vi "fix_ICS_msg.vi"(11 "Msg in":string) -> (3 "JSON":string)   [LabVIEW 2018]
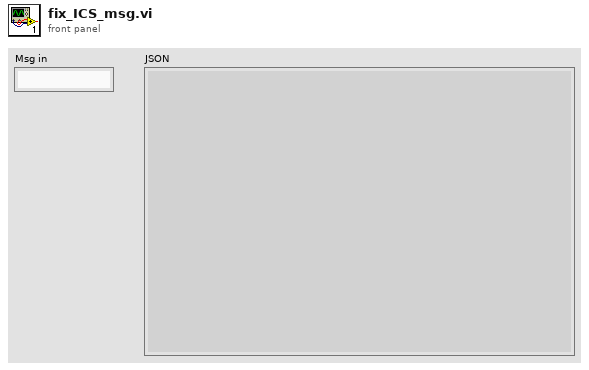
[diagram p1: front panel]
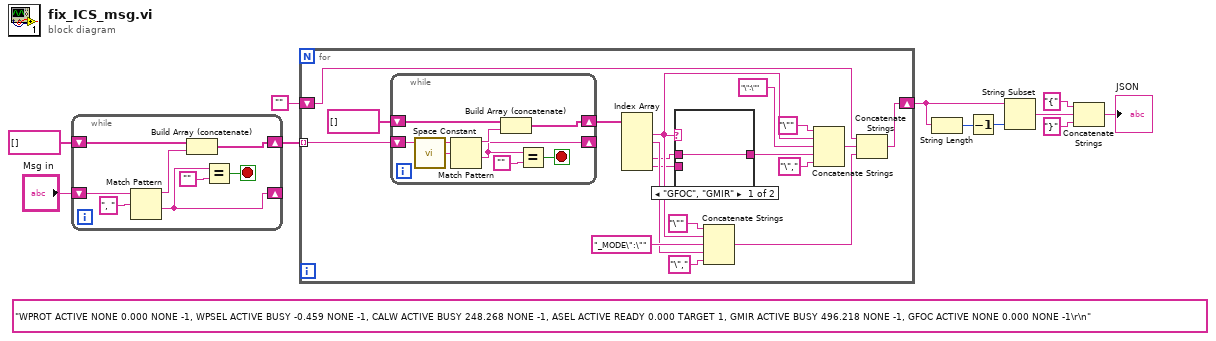
[diagram p0: block diagram]
diagram:
  (unwired) "WPROT ACTIVE NONE 0.000 NONE -1, WPSEL ACTIVE BUSY -0.459 NONE -1, CALW ACTIVE BUSY 248.268 NONE -1, ASEL ACTIVE READY 0.000 TARGET 1, GMIR ACTIVE BUSY 496.218 NONE -1, GFOC ACTIVE NONE 0.000 NONE -1\r\n" ("search string/char (-)")
  n1 = while {
    shift-right: [w16] -> w2
    shift-left: string[] [] -> [w17]
    shift-right: [w12] -> _
    shift-left: "Msg in" -> [w15]
    stop <- w18 stop-if-true
    n2 = Match Pattern(string=w15, regular expression=", " ("search string/char (-)")) -> (before substring=w13:string, after substring=w12:string)  [unwired: 1 in, 2 out]
    n3 = Build Array (concatenate)(w17, w13) -> (w16:string[])
    n4 = Equal?(x=w12, y="") -> (x = y?=w18:bool)
  }
  n5 = for {
    tunnel: w2 -> [w36] mode=indexing
    shift-right: [w25] -> w4
    shift-left: "" -> [w24]
    n6 = while {
      shift-right: [w44] -> w35
      shift-left: string[] [] -> [w45]
      shift-right: [w41] -> _
      shift-left: w36 -> [w43]
      stop <- w46 stop-if-true
      n7 = call <vilib>:"Space Constant.vi"() -> ("String"=w40:string)
      n8 = Match Pattern(string=w43, regular expression=w40) -> (before substring=w42:string, after substring=w41:string)  [unwired: 1 in, 2 out]
      n9 = Build Array (concatenate)(w45, w42) -> (w44:string[])
      n10 = Equal?(x=w41, y="") -> (x = y?=w46:bool)
    }
    n11 = Index Array(array=w35) -> (element #1=w22:string, element #2=w28:string, element #4=w20:string, element #5=w21:string)  [unwired: 5 in, 1 out]
    n12 = case shown="\"GFOC\", \"GMIR\"" w22 {
      tunnel: [w38 w39] -> w23
      tunnel: w21 -> [_ w39]
      tunnel: w20 -> [w38 _]
      frame "GFOC", "GMIR" {
      }
      frame "True", Default {
      }
    }
    n13 = Concatenate Strings("\"" ("search string/char (-)"), w22, "_MODE\":\"" ("search string/char (-)"), w28, "\"," ("search string/char (-)")) -> (w27:string)
    n14 = Concatenate Strings("\"" ("search string/char (-)"), w22, "\":\"" ("search string/char (-)"), w23, "\"," ("search string/char (-)")) -> (w26:string)
    n15 = Concatenate Strings(w24, w26, w27) -> (w25:string)
  }
  n16 = String Length(string=w4) -> (length=w6:i32)
  n17 = Decrement(x=w6) -> (x-1=w5:i32)
  n18 = String Subset(string=w4, length (rest)=w5) -> (substring=w7:string)  [unwired: 1 in]
  n19 = Concatenate Strings("{" ("search string/char (-)"), w7, "}" ("search string/char (-)")) -> (→"JSON":string)
